vi "Action.vi"(8 "error in (no error)":errorcluster, 10 "Action":string, 11 "HarnessInterface in":refnum<class "PluginHarness.lvclass">) -> (0 "error out":errorcluster, 3 "HarnessInterface out":refnum<class "PluginHarness.lvclass">)   [LabVIEW 2021, in "PluginHarness.lvlib" / "PluginHarness.lvclass"]
uses:
  PluginHarness.lvclass
  PluginHarness.lvclass/PluginHarness.ctl
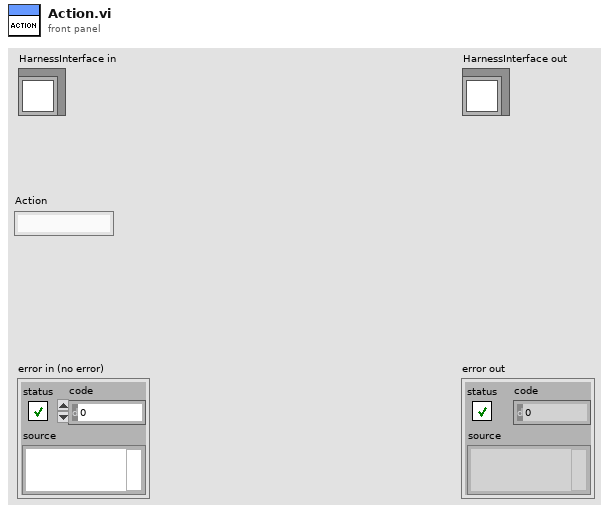
[diagram p1: front panel]
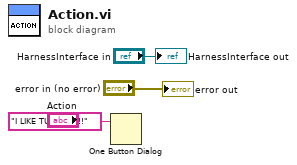
[diagram p0: block diagram]
diagram:
  n1 = One Button Dialog(message="I LIKE TURTLES!!!") -> ()  [unwired: 1 in, 1 out]
  "error out" <- "error in (no error)"
  "HarnessInterface out" <- "HarnessInterface in"
